vi "LVClass_CorrectionDataManager GetCorrectionMode.vi"(0 "CorrectionDataManager in":refnum<class "CorrectionDataManager.lvclass">, 11 "error in (no error)":errorcluster) -> (4 "CorrectionDataManager out":refnum<class "CorrectionDataManager.lvclass">, 6 "Use Phase?":bool, 15 "error out":errorcluster)   [LabVIEW 2020, in "CorrectionDataManager.lvclass"]
doc: "Get correction data manager type (Slopes or Phase type)\n\n<B>corrdata_managerIn</B> : CorrDataManager object.\n<B>corrdata_managerOut</B> : CorrDataManager object.\n<B>is_phase</B> : define if influence container is a HasoSlopes or Phase."
uses:
  CorrectionDataManager.lvclass
  CorrectionDataManager.lvclass/CorrectionDataManager.ctl
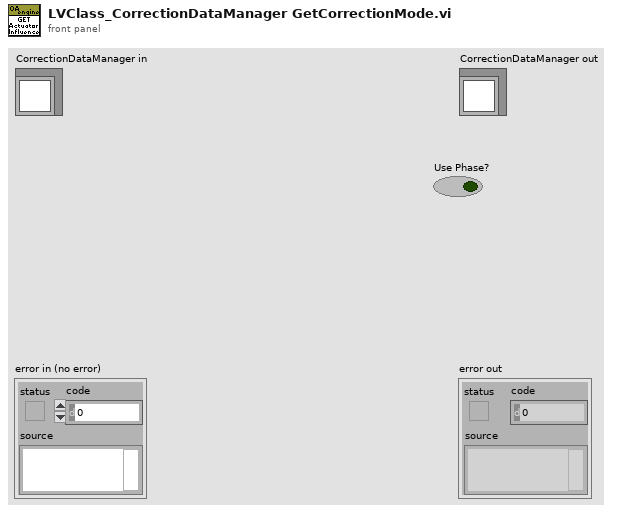
[diagram p1: front panel]
types:
  T1 = typedef "ClassID.ctl" = i64
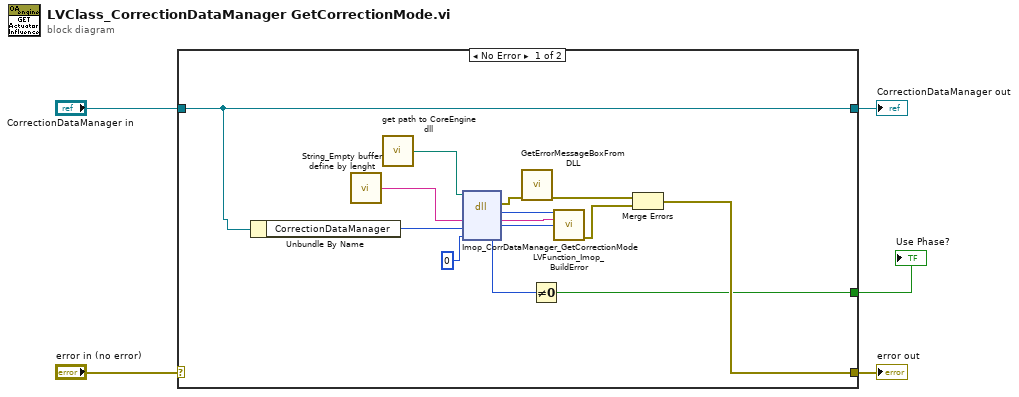
[diagram p0: block diagram]
diagram:
  n1 = case shown="No Error" "error in (no error)" {
    selector: "error in (no error)" -> [_ w21]
    tunnel: [w12 w21] -> w5
    tunnel: [w10 w20] -> w4
    tunnel: "CorrectionDataManager in" -> [w10 w20]
    tunnel: [w7 _] -> w1
    frame No Error {
      n2 = Unbundle By Name(w10) -> ("CorrectionDataManager"=w11:T1)
      n3 = call "String_Empty buffer define by lenght.vi"() -> ("Empty buffer"=w17:string)  [unwired: 1 in]
      n4 = call "get path to CoreEngine dll.vi"() -> ("path to wavekit library"=w16:path)  [unwired: 14 in, 1 out]
      n5 = dll-call lib="D:/FLE/0.Code/CoreEngine4_Suite/LV2011_interface/DLLs/c_interface_vc100.dll" fn="Imop_CorrDataManager_GetCorrectionMode"(path in=w16, "message"=w17, "corrdata_manager"=w11, "use phase"=u8 0) -> (error out=w15:errorcluster, "return type"=w19:i32, "message"=w18:string, "corrdata_manager"=w6:i64, "use phase"=w8:u8)  [unwired: 2 in, 1 out]
      n6 = call "GetErrorMessageBoxFromDLL.vi"("error IN"=w15) -> ("error OUT"=w14:errorcluster)  [unwired: 10 in]
      n7 = Not Equal To 0?(x=w8) -> (x != 0?=w7:bool)
      n8 = call "LVFunction_Imop_BuildError.vi"("code"=w19, "String to Prepend to source (\"\")"=w18, "Adresse"=w6) -> ("error out"=w13:errorcluster)  [unwired: 12 in]
      n9 = Merge Errors(w14, w13) -> (w12:errorcluster)
    }
    frame Error {
    }
  }
  "error out" <- w5
  "CorrectionDataManager out" <- w4
  "Use Phase?" <- w1
